vi "Configure Timing.vi"(1 "External  Reference Clock Option":u16(ring) items=["Frequency Value", "Default", "Minimum", "Maximum"], 2 "Sampling Clock Option":u16(ring) items=["Frequency Value", "Default", "Minimum", "Maximum"], 4 "External Reference Clock (Hz)":dbl format="%#_16g", 5 "error in (no error)":errorcluster, 6 "Sampling Clock (Hz)":dbl format="%#_16g", 7 "Clock Source":u16(ring) items=["Internal", "External"], 8 "VISA resource name":refnum<visa-resource-name>) -> (0 "error out":errorcluster, 3 "VISA resource name out":refnum<visa-resource-name>)   [LabVIEW 2020, in "Active Technologies AWG3000.lvlib"]
uses:
  Active Technologies AWG3000.lvlib
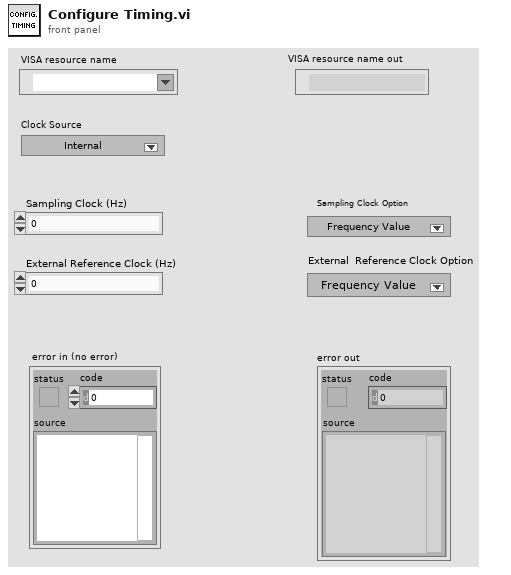
[diagram p1: front panel]
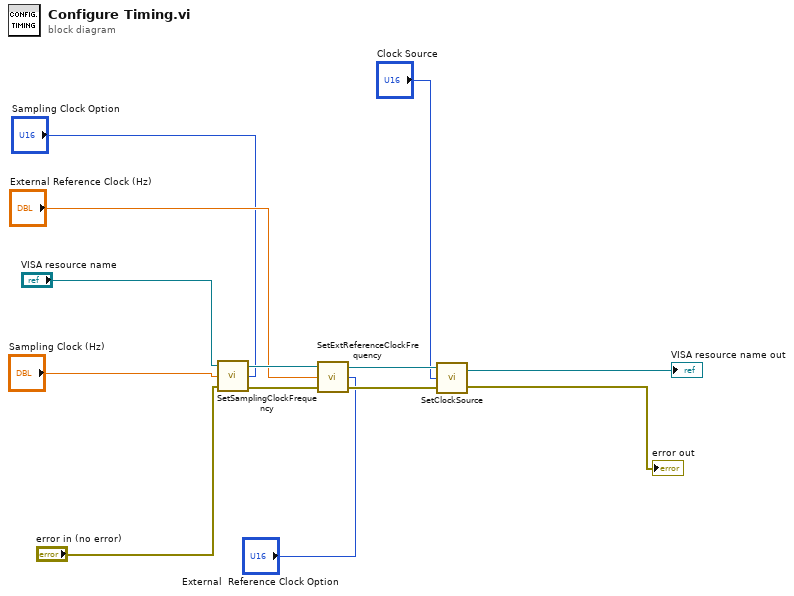
[diagram p0: block diagram]
diagram:
  n1 = call "SetSamplingClockFrequency.vi"("Sampling Clock Option"="Sampling Clock Option", "error in (no error)"="error in (no error)", "Sampling Clock (Hz)"="Sampling Clock (Hz)", "VISA resource name"="VISA resource name") -> ("error out"=w9:errorcluster, "VISA resource name out"=w10:refnum<visa-resource-name>)
  n2 = call "SetExtReferenceClockFrequency.vi"("External  Reference Clock Option"="External  Reference Clock Option", "error in (no error)"=w9, "External Reference Clock (Hz)"="External Reference Clock (Hz)", "VISA resource name"=w10) -> ("error out"=w8:errorcluster, "VISA resource name out"=w5:refnum<visa-resource-name>)
  n3 = call "SetClockSource.vi"("error in (no error)"=w8, "Clock Source"="Clock Source", "VISA resource name"=w5) -> ("error out"=→"error out":errorcluster, "VISA resource name out"=→"VISA resource name out":refnum<visa-resource-name>)
